vi "Simulate_kernal.vi"() -> (0 "error out":errorcluster)   [LabVIEW 2022 SP3]
uses:
  Sub_vis/Upload Data.ctl
  Globals/Meas_global.vi
  Globals/Trav_pos_global.vi
  <vilib>/Analysis/NI_AALBase.lvlib
panel:
  in  "No Of samples":dbl
  in  "Instrument freq":dbl=30.0
  in  "Max Peak":dbl=1.0
  out "Waveform Graph":dbl[][](graph)
  in  "Random?":bool
  in  "Average Value":dbl
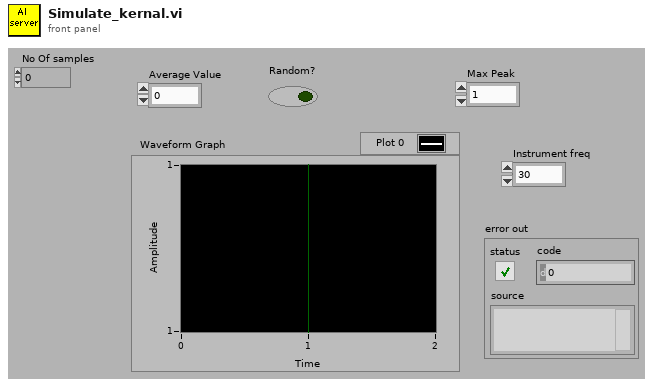
[diagram p1: front panel]
types:
  T1 = typedef "Setup.ctl" = enum16{"Run Program", "Show Setup", "Save Current Setup", "Setup Front Panel"}
  T2 = typedef "Upload Data.ctl" = enum16{"Voltage Array", "Time Trace Cluster"}
  T3 = typedef "Analysis_info_cluster.ctl" = cluster{"Colour":u32, "Inst type":T4, "Inst name":string, "Symbol":string, "Code name":string, "Extra Info":string, "Inst Array":T5, "Extra Titles":string[], "Extra Values":string[], "U":dbl, "u^2":dbl, "u^3":dbl, "u^4":dbl, "Skew_u":dbl, "Kurt_u":dbl, "Sd Error in Mean":dbl, "% u'/U":dbl, "X":dbl, "Y":dbl, "Z":dbl, "Timescale integral Estimate":dbl, "Sd Error in Variance":dbl, "Calib File":path, "Calib Constants":dbl[], "Output Position":bool, "Stats":enum16{"None", "Basic", "Full"}, "Av Sampling Rate":dbl, "Av No of Samples":dbl, "Total Meas Time (s)":dbl, "ADAM Ch Name":string, "Max value":dbl, "Min value":dbl, "Req Sample Rate Hz":dbl, "Sync Delay Time (s)":dbl, "Ch No":i16, "Device":string, "Use Latest Calib":bool, "Port":string, "Metadata Ch Names":string[], "Metadata Ch Values":string[], "Label":string}
  T4 = typedef "Inst_type.ctl" = enum16{"Raw voltage", "Raw with zero offsetting", "Propeller anemometer", "Pressure Transducer", "Pitot-static tube", "Hot wire", "Cross wire 1", "Cross wire 2", "Generic Linear", "Generic Polynomial", "Generic BackPoly", "Fast FID", "Thermocouple", "Cold wire", "Pulsed Wire", "LDA Vel", "LDA Tran time", "LDA Arr time", "Microphone"}
  T5 = typedef "Instrument_Array.ctl" = enum16{"PWA", "LDA", "Analogue"}
  T6 = typedef "Rendezvous RefNum" = refnum<k1>
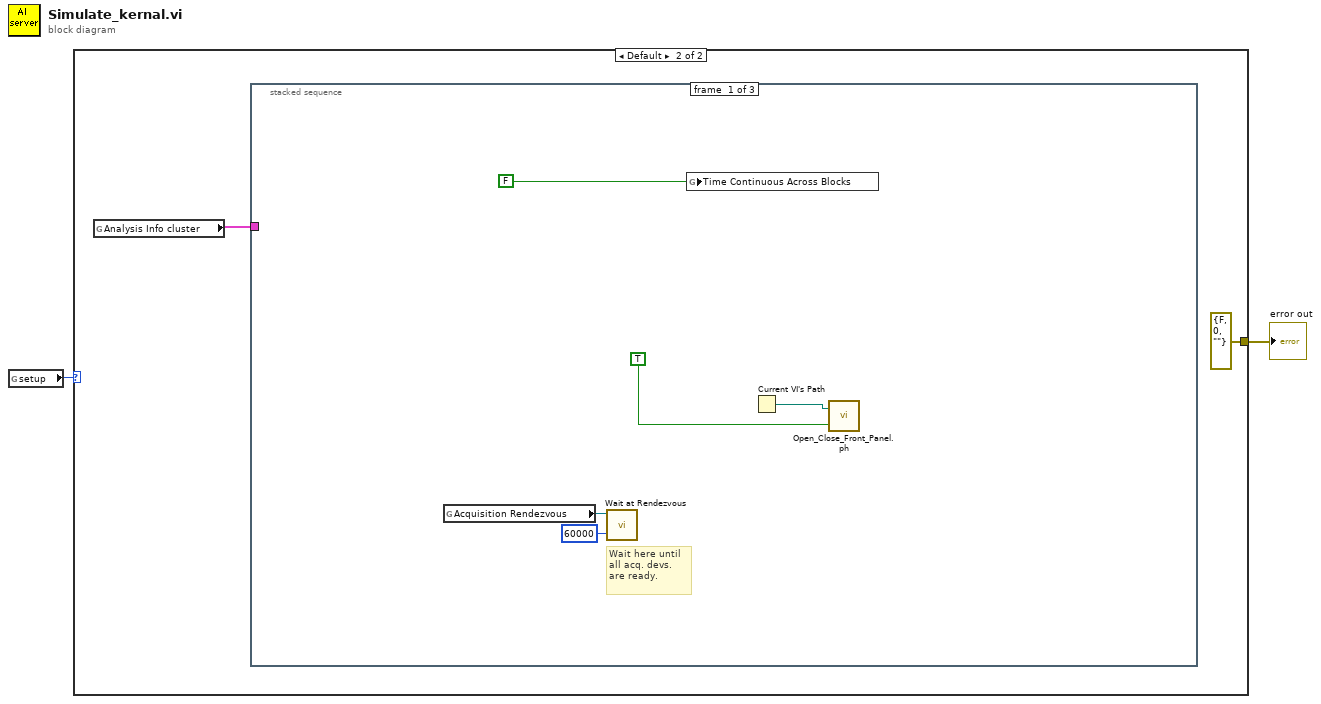
[diagram p0: block diagram]
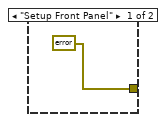
[diagram p2: hidden frame]
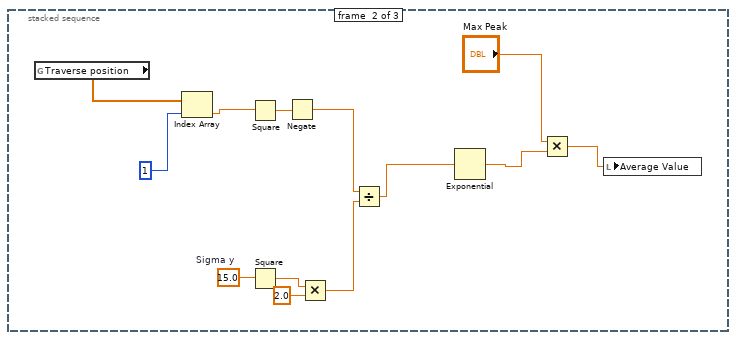
[diagram p3: hidden frame]
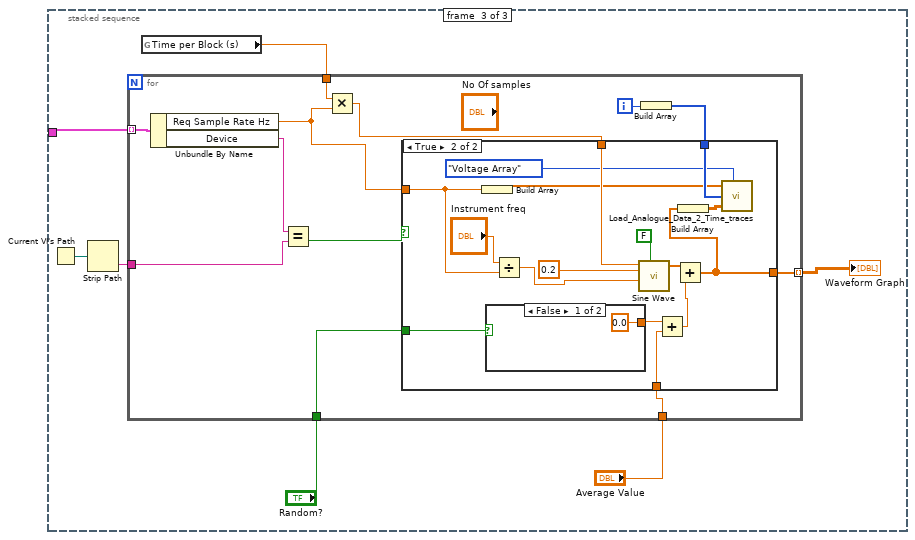
[diagram p4: hidden frame]
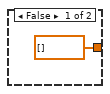
[diagram p5: hidden frame]
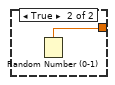
[diagram p6: hidden frame]
diagram:
  n1 = global read "Meas_global.vi" "setup"() -> (w2:T1)
  n2 = case shown="Default" w2 {
    tunnel: [errorcluster {"status"=FALSE, "code"=0, "source"=""} ("error out") errorcluster {"status"=FALSE, "code"=0, "source"=""} ("error out")] -> w1
    frame "Setup Front Panel" {
    }
    frame Default {
      n3 = global read "Meas_global.vi" "Analysis Info cluster"() -> (w5:T3[])
      n4 = stacked-sequence {
        tunnel: w5 -> [_ _ w27]
        frame #0 {
          # "Wait here until all acq. devs. are ready."
          n5 = global read "Meas_global.vi" "Acquisition Rendezvous"() -> (w7:T6)
          n6 = call <vilib>:"Wait at Rendezvous.vi"("ms timeout (-1)"=60000, "rendezvous"=w7) -> ()  [unwired: 3 in, 3 out]
          n7 = global write "Meas_global.vi" "Time Continuous Across Blocks"(FALSE ("Time Continuous across Blocks")) -> ()
          n8 = Current VI's Path() -> (path=w10:path)
          n9 = call "Open_Close_Front_Panel.ph.vi"("openWindow (T)"=TRUE ("Front Panel Window:Open"), "VI path"=w10) -> ()  [unwired: 1 in, 1 out]
        }
        frame #1 {
          w19 = 15.0  # Sigma y
          n10 = global read "Trav_pos_global.vi" "Traverse position"() -> (w23:sgl[])
          n11 = Index Array(array=w23, index=1) -> (element=w21:sgl)
          n12 = Square(x=w21) -> (x^2=w20:sgl)
          n13 = Square(x=w19) -> (x^2=w18:dbl)
          n14 = Negate(x=w20) -> (-x=w16:sgl)
          n15 = Multiply(x=w18, y=2.0) -> (x*y=w15:dbl)
          n16 = Divide(x=w16, y=w15) -> (x/y=w14:dbl)
          n17 = Exponential(1:w14) -> (0:w13:dbl)
          n18 = Multiply(x="Max Peak", y=w13) -> (x*y=w11:dbl)
          n19 = local write "Average Value"(w11) -> ()
        }
        frame #2 {
          n20 = Current VI's Path() -> (path=w25:path)
          n21 = Strip Path(path=w25) -> (name=w24:string)  [unwired: 1 out]
          n22 = global read "Meas_global.vi" "Time per Block (s)"() -> (w26:dbl)
          n23 = for {
            tunnel: [w38] -> w28 mode=indexing
            tunnel: "Random?" -> [w42]
            tunnel: "Average Value" -> [w41]
            tunnel: w27 -> [w40] mode=indexing
            tunnel: w26 -> [w39]
            tunnel: w24 -> [w36]
            i -> [w34]
            n24 = Unbundle By Name(w40) -> ("Req Sample Rate Hz"=w32:dbl, "Device"=w37:string)
            n25 = Equal?(x=w37, y=w36) -> (x = y?=w35:bool)
            n26 = Multiply(x=w39, y=w32) -> (x*y=w31:dbl)
            n27 = Build Array(w34) -> (w33:i32[])
            n28 = case shown="True" w35 {
              tunnel: w42 -> [_ w57]
              tunnel: w41 -> [_ w54]
              tunnel: w31 -> [_ w52]
              tunnel: [dbl[] [] w49] -> w38
              tunnel: w33 -> [_ w51]
              tunnel: w32 -> [_ w46]
              frame False {
              }
              frame True {
                n29 = Build Array(w46) -> (w50:dbl[])
                n30 = case shown="False" w57 {
                  tunnel: [0.0 ("number: 0 to 1") w61] -> w56
                  frame False {
                  }
                  frame True {
                    n31 = Random Number (0-1)() -> (number: 0 to 1=w61:dbl)
                  }
                }
                n32 = Divide(x="Instrument freq", y=w46) -> (x/y=w45:dbl)
                n33 = call <vilib>:"Sine Wave.vi"("samples"=w52, "amplitude"=0.2, "frequency"=w45, "reset phase"=FALSE) -> ("sine wave"=w59:dbl[])  [unwired: 1 in, 2 out]
                n34 = Add(x=w56, y=w54) -> (x+y=w55:dbl)
                n35 = Add(x=w59, y=w55) -> (x+y=w49:dbl[])
                n36 = Build Array(w49) -> (w48:dbl[][])
                n37 = call "Load_Analogue_Data_2_Time_traces.vi"("Sampling Rate (Hz)"=w50, "Mode"=Upload_Data."Voltage Array", "Index"=w51, "Voltage Array"=w48) -> ()  [unwired: 3 in]
              }
            }
          }
          "Waveform Graph" <- w28
        }
      }
    }
  }
  "error out" <- w1
